vi "route finding algorithm basic.vi"() -> ()   [LabVIEW 2015]
uses:
  <vilib>/Platform/TimedLoop/XDataNode/timing_clust.ctl
  <vilib>/Platform/TimedLoop/XDataNode/nitl_modes.ctl
  <vilib>/Platform/TimedLoop/XDataNode/wakeup.ctl
  <vilib>/Platform/TimedLoop/XDataNode/XDataNode.xnode
  <vilib>/robotics/Navigation/shared/WorldMap/OccupancyGridWorldMap/NI_Robotics_OccupancyGridWorldMap.lvclass
  <vilib>/robotics/Navigation/NI_Robotics_Navigation .lvlib
  <vilib>/Platform/TimedLoop/XDataNode/XDNodeRunTimeDep.lvlib
panel:
  out "Map":u16[][](array[ring])
  in  "stop":bool
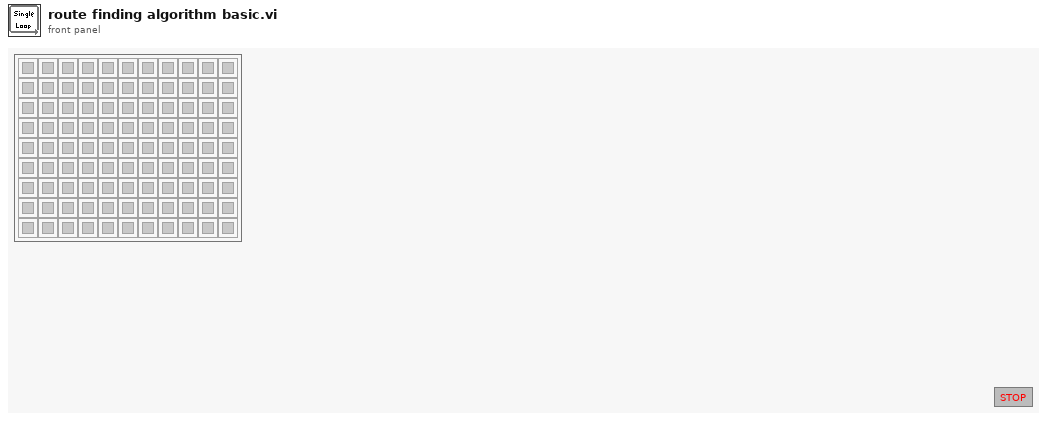
[diagram p1: front panel]
types:
  T1 = typedef "XDNodeRunTimeDep.lvlib/timing_clust.ctl" = cluster{"Expected End [f-1]":u64, "Actual End [f-1]":u64, "Finished Late? [f-1]":bool, "Expected End [i-1]":u64, "Actual End [i-1]":u64, "Finished Late? [i-1]":bool, "Expected Start [i]":u64, "Actual Start [i]":u64, "Expected Start [f]":u64, "Actual Start [f]":u64, "Source Name":string, "Structure Name":string, "Period":i64, "Deadline":i64, "Offset":i64, "Start":i64, "Priority":i32, "Timeout":i32, "Mode":T2, "Wakeup Reason":T3, "Error":errorcluster, "Source Type":string, "Secondary Source Type":string, "Global End Time":u64, "Global Start Time":u64, "Frame Duration":u64, "Iteration Duration":u64, "Assigned CPU":i32, "I/O Scan Engine Mode":u32}
  T2 = typedef "XDNodeRunTimeDep.lvlib/nitl_modes.ctl" = enum32{"No Change", "Process missed periods, maintain original phase", "Discard missed periods, maintain original phase", "Process missed periods, ignore original phase", "Discard missed periods, ignore original phase"}
  T3 = typedef "XDNodeRunTimeDep.lvlib/wakeup.ctl" = enum32{"Normal", "Aborted", "Asynchronous wakeup", "Timing source error", "Timed loop error", "Timeout"}
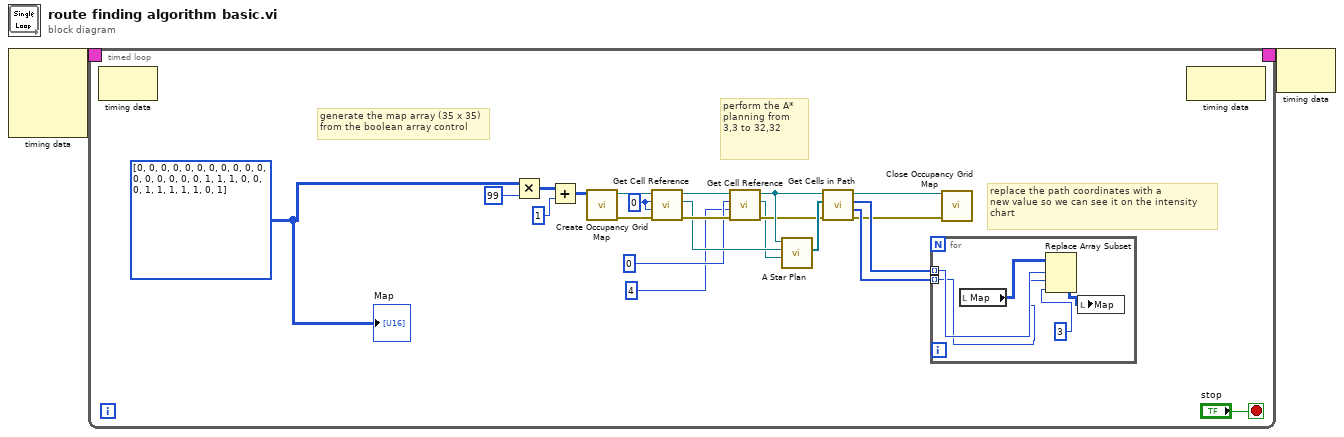
[diagram p0: block diagram]
diagram:
  n1 = node-c288() -> (w2:T1)  [unwired: 4 in]
  n2 = timed-loop {
    timing: w2 -> [_]
    timing-out: [_] -> w1
    stop <- "stop" stop-if-true
    w3 = i32[][] [[0, 0, 0, 0, 0, 0], [0, 0, 0, 0, 0, 0], [0, 0, 0, 0, 0, 1], [1, 1, 0, 0, 0, 1], [1, 1, 1, 1, 0, 1]]
    w21 = 0 ("x")
    # "replace the path coordinates with a\nnew value so we can see it on the intensity \nchart"
    # "perform the A* planning from 3,3 to 32,32"
    # "generate the map array (35 x 35)\nfrom the boolean array control"
    n3 = node-c288() -> ()  [unwired: 1 in, 1 out]
    n4 = Multiply(x=w3, y=99) -> (x*y=w17:i32[][])
    n5 = Add(x=w17, y=1) -> (x+y=w15:i32[][])
    n6 = call <vilib>:"Create Occupancy Grid Map.vi"("occupancy grid"=w15) -> ("error out"=w14:errorcluster, "map reference out"=w10:refnum<data-value>)  [unwired: 9 in]
    n7 = call <vilib>:"Get Cell Reference.vi"("error in (no error)"=w14, "y"=w21, "x"=w21, "map reference in"=w10) -> ("error out"=w13:errorcluster, "cell reference"=w11:refnum<data-value>, "map reference out"=w24:refnum<data-value>)  [unwired: 4 in, 1 out]
    n8 = call <vilib>:"Get Cell Reference.vi"("error in (no error)"=w13, "y"=4, "x"=0, "map reference in"=w24) -> ("error out"=w12:errorcluster, "cell reference"=w9:refnum<data-value>, "map reference out"=w22:refnum<data-value>)  [unwired: 4 in, 1 out]
    n9 = call <vilib>:"A Star Plan.vi"("goal reference"=w9, "start reference"=w11, "map reference in"=w22) -> ("path references"=w23:refnum<data-value>[])  [unwired: 5 in, 3 out]
    n10 = call <vilib>:"Get Cells in Path.vi"("error in (no error)"=w12, "path references"=w23, "map reference in"=w22) -> ("error out"=w4:errorcluster, "y coordinates"=w20:i32[], "x coordinates"=w19:i32[], "map reference out"=w5:refnum<data-value>)  [unwired: 5 in]
    n11 = for {
      tunnel: w20 -> [w29] mode=indexing
      tunnel: w19 -> [w30] mode=indexing
      n12 = local read "Map"() -> (w31:u16[][])
      n13 = Replace Array Subset(array=w31, new element=3, index (row)=w30, index (col)=w29) -> (w28:u16[][])
      n14 = local write "Map"(w28) -> ()
    }
    n15 = call <vilib>:"Close Occupancy Grid Map.vi"("error in (no error)"=w4, "map reference in"=w5) -> ()  [unwired: 9 in, 1 out]
    n16 = node-c288() -> ()  [unwired: 1 in, 1 out]
    "Map" <- w3
  }
  n17 = node-c288(w1) -> ()  [unwired: 1 out]
